vi "Set-application-path.vi"(8 "error in (no error)":errorcluster, 10 "Main VI ref":refnum<vi>, 11 "Data ref. in":refnum<data-value>) -> (0 "error out":errorcluster, 3 "Data ref.":refnum<data-value>)   [LabVIEW 2013, in "CameraVision.lvlib" / "CV-Main.lvclass"]
uses:
  CV-Main.lvclass
  CV-Main.lvclass/CV-Main.ctl
  Storage/CV-Storage.lvclass/CV-Storage.ctl
  Read Storage params.vi
  Storage/Write Base path.vi
  Storage/CV-Storage.lvclass
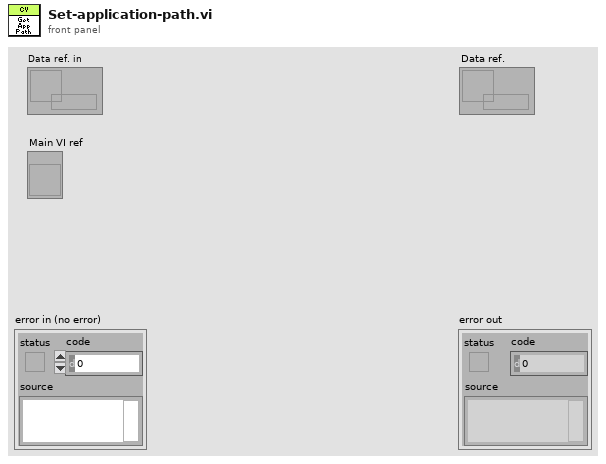
[diagram p1: front panel]
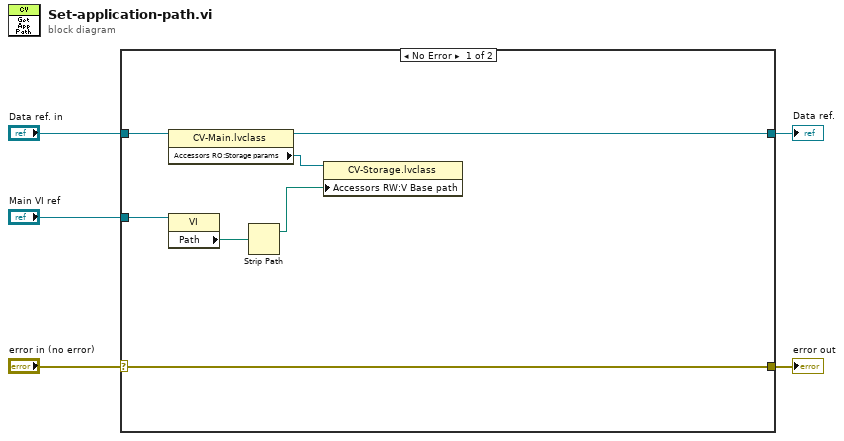
[diagram p0: block diagram]
diagram:
  n1 = case shown="No Error" "error in (no error)" {
    selector: "error in (no error)" -> [w11 w14]
    tunnel: [w11 w14] -> w4
    tunnel: "Data ref. in" -> [w12 w13]
    tunnel: [w10 w13] -> w2
    tunnel: "Main VI ref" -> [w8 _]
    frame No Error {
      n2 = property class="CV-Main.lvclass"(reference=w12) -> (reference out=w10:refnum<data-value>, "Accessors RO:Storage params"=w9:refnum<data-value>)  [unwired: 1 in, 1 out]
      n3 = property class="VI"(reference=w8) -> ("Path"=w7:path)  [unwired: 1 in, 2 out]
      n4 = Strip Path(path=w7) -> (stripped path=w6:path)  [unwired: 1 out]
      n5 = property class="CV-Storage.lvclass"(reference=w9, "Accessors RW:V Base path"=w6) -> ()  [unwired: 1 in, 2 out]
    }
    frame Error {
    }
  }
  "error out" <- w4
  "Data ref." <- w2
